vi "ObtainQueue.vi"(7 "Destroy? (f)":bool, 8 "ErrorArray":errorcluster[](array[cluster])) -> (0 "ErrorArray.":errorcluster[](array[cluster]), 3 "TstQue":refnum<queue>)   [LabVIEW 2014, in "TestBase.lvclass"]
uses:
  TestBase.lvclass
  clQueMsgType.ctl
  <userlib>/NIST/NISTErrorLib/NISTErrorLib.lvlib
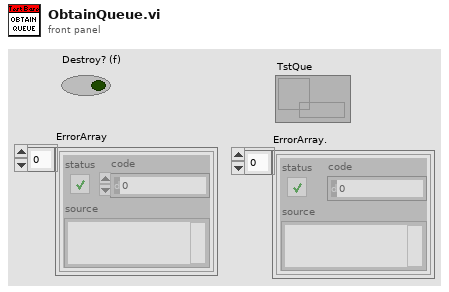
[diagram p1: front panel]
types:
  T1 = typedef "TestBase.lvclass/clQueMsgType.ctl" = cluster{"Message":string, "Data":variant}
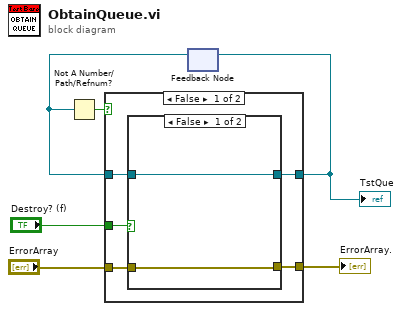
[diagram p0: block diagram]
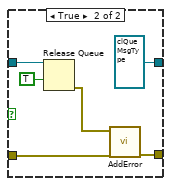
[diagram p2: hidden frame]
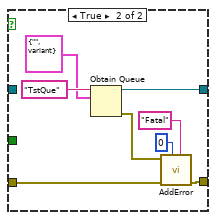
[diagram p3: hidden frame]
diagram:
  n1 = feedback #1() -> (w2:refnum<queue>)  [unwired: 1 in]
  n2 = Not A Number/Path/Refnum?(number/path/refnum=w2) -> (NaN/Path/Refnum?=w3:bool)
  n3 = case shown="False" w3 {
    tunnel: [w8 w24] -> w6
    tunnel: "ErrorArray" -> [w7 w21]
    tunnel: [w9 w20] -> w4
    tunnel: w2 -> [w11 _]
    tunnel: "Destroy? (f)" -> [w10 _]
    frame False {
      n4 = case shown="False" w10 {
        tunnel: w11 -> [w13 w19]
        tunnel: [w13 refnum<queue> refnum ("queue out")] -> w9
        tunnel: [w12 w17] -> w8
        tunnel: w7 -> [w12 w16]
        frame False {
        }
        frame True {
          n5 = Release Queue(queue=w19, force destroy? (F)=TRUE) -> (error out=w15:errorcluster)  [unwired: 1 in, 2 out]
          n6 = call <userlib>:"AddError.vi"("ErrorArray"=w16, "error in (no error)"=w15) -> ("ErrorArray"=w17:errorcluster[])  [unwired: 8 in, 1 out]
        }
      }
    }
    frame True {
      n7 = Obtain Queue(name (unnamed)="TstQue", element data type=T1 {"Message"="", "Data"=variant} ("clQueMsgType")) -> (queue out=w20:refnum<queue>, error out=w25:errorcluster)  [unwired: 3 in, 1 out]
      n8 = call <userlib>:"AddError.vi"("Severity"="Fatal", "Priority"=u8 0, "ErrorArray"=w21, "error in (no error)"=w25) -> ("ErrorArray"=w24:errorcluster[])  [unwired: 6 in, 1 out]
    }
  }
  "ErrorArray." <- w6
  "TstQue" <- w4
  n9 = feedback-in #1(w4) -> ()
